vi "Set miniscan point numerical entry limits.vi"(8 "error in":errorcluster, 10 "Properties of selected ROI":cluster{"Type":T1, "Points per cycle":u16}) -> (0 "error out":errorcluster)   [LabVIEW 2013]
uses:
  xcontrol/Interface VIs/Interface typedefs/Interface-ROI type enum.ctl
  Global variables/gl_Functional Imaging-Global variables.vi
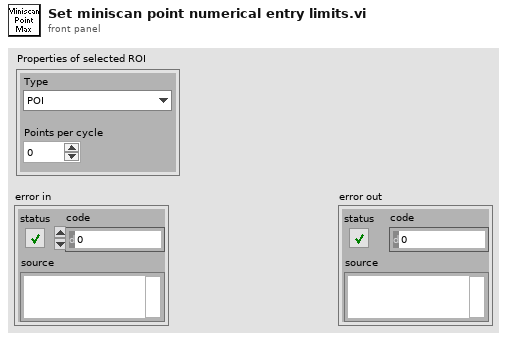
[diagram p1: front panel]
types:
  T1 = typedef "Interface-ROI type enum.ctl" = enum16{"POI", "Mini-scan"}
  T2 = typedef "Functional Imging UI Refs.ctl" = cluster{"Menu ref":refnum<k9>, "Image control":refnum<vi>, "VI ref":refnum<vi>, "XGrapher":refnum<vi>, "Smoothing":refnum<vi>, "POI Averaging":refnum<vi>, "Normalize":refnum<vi>, "POI data points in each trial":refnum<vi>, "Channel":refnum<vi>, "Experiment data folder path":refnum<vi>, "[ROI vis]":refnum<vi>, "[Groups] visbl":T3, "Group Name":refnum<vi>, "POI index":refnum<vi>, "Trial No.":refnum<vi>, "Intensity Zoom":refnum<vi>, "Trial Cursor Enabled":refnum<vi>, "Number of Trials (ind 1)":refnum<vi>, "Number of Trials (ind 2)":refnum<vi>, "MiniScans Available":refnum<vi>, "POI Available":refnum<vi>, "Defer graph updates":refnum<vi>, "Waveform selector":refnum<vi>, "#of selected POI":refnum<vi>, "#of selected MiniScans":refnum<vi>, "#of selected groups":refnum<vi>, "Max Z-Projection":refnum<vi>, "Z-Plane Selector":refnum<vi>, "Index of miniscan point to visualise":refnum<vi>, "ROI vis. mode":refnum<vi>, "Total # of points":refnum<vi>, "Index of group clicked on":refnum<vi>, "Pane 1":refnum<vi>, "Pane 2":refnum<vi>, "Pane 3":refnum<vi>, "Pane 4":refnum<vi>, "Pane 5":refnum<vi>, "Pane 6":refnum<vi>, "Deselect all ROI":refnum<vi>, "Deselect all groups":refnum<vi>}
  T3 = typedef "Groups array referecne.ctl" = refnum<vi>
  T4 = enum8{"Enabled", "Disabled", "Disabled and Grayed Out"}
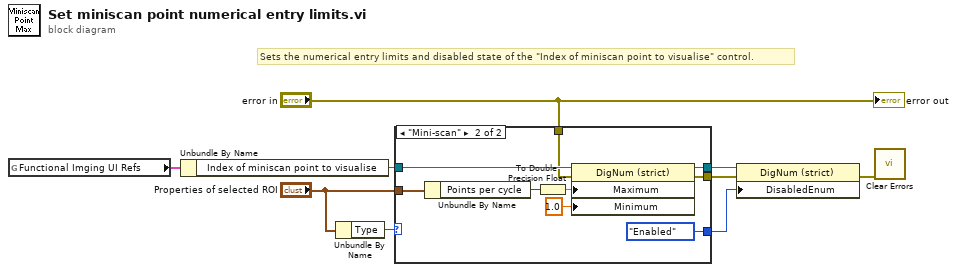
[diagram p0: block diagram]
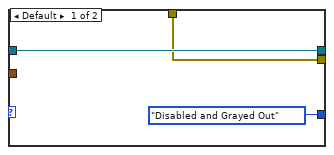
[diagram p2: hidden frame]
diagram:
  # "Sets the numerical entry limits and disabled state of the \"Index of miniscan point to visualise\" control."
  n1 = global read "gl_Functional Imaging-Global variables.vi" "Functional Imging UI Refs"() -> (w3:T2)
  n2 = Unbundle By Name(w3) -> ("Index of miniscan point to visualise"=w9:refnum<vi>)
  n3 = Unbundle By Name("Properties of selected ROI") -> ("Type"=w2:T1)
  n4 = case shown="\"Mini-scan\"" w2 {
    tunnel: w9 -> [w12 w19]
    tunnel: "error in" -> [w10 w18]
    tunnel: "Properties of selected ROI" -> [_ w17]
    tunnel: [w12 w16] -> w7
    tunnel: [T4."Disabled and Grayed Out" ("Disabled") T4."Enabled" ("Disabled")] -> w6
    tunnel: [w10 w15] -> w5
    frame Default {
    }
    frame "Mini-scan" {
      n5 = Unbundle By Name(w17) -> ("Points per cycle"=w20:u16)
      n6 = To Double Precision Float(number=w20) -> (double precision float=w13:dbl)
      n7 = property on="Property Node" class="DigNum (strict)"(reference=w19, error in=w18, "Maximum"=w13, "Minimum"=1.0 ("Data Entry Limits:Minimum")) -> (reference out=w16:refnum<vi>, error out=w15:errorcluster)
    }
  }
  n8 = property on="Property Node" class="DigNum (strict)"(reference=w7, error in=w5, "DisabledEnum"=w6) -> (error out=w4:errorcluster)  [unwired: 1 out]
  n9 = call <vilib>:"Clear Errors.vi"("error in (no error)"=w4) -> ()  [unwired: 6 in, 1 out]
  "error out" <- "error in"
